vi "setposition.vi"(1 "Vy":dbl, 2 "Vx":dbl) -> ()   [LabVIEW 2015]
uses:
  <vilib>/DAQmx/write.llb/DAQmx Write (Analog 1D DBL NChan 1Samp).vi
  <vilib>/DAQmx/create/channels.llb/DAQmx Create Channel (AO-Voltage-Basic).vi
  <vilib>/DAQmx/miscellaneous.llb/DAQmx Fill In Error Info.vi
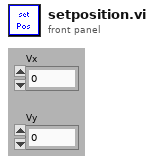
[diagram p1: front panel]
types:
  T1 = typedef "XYZStage.lvlib/XYZStage Configuration.ctl" = cluster{"VISA resource name":refnum<visa-resource-name>, "Timeout (3sec)":u32}
  T2 = cluster{"StageS":i32, "StageL":i32, "currmeas data dir":path, "image OD":u16, "contour OD":u16, "point OD":u16, "AOlines":tag[], "AIlines":tag[], "CI lines":tag[], "DO lines":tag[], "AO names":string[], "CI names":string[], "AI names":string[], "DO names":string[], "CIextensions":string[], "AIextensions":string[], "Voltage to Ygalvo":i32, "Voltage to Xgalvo":i32, "Voltage to patch":i32, "640 shutter":i32, "2P shutter":i32, "LT timestamp":u32, "Vp":i32, "Ip":i32, "camera trigger":i32, "master data dir":path, "voltage to Zpos":i32, "Vto2P":i32, "640 AO":i32, "488 AO":i32, "532 AO":i32, "640TTL":u32, "488TTL":u32, "532TTL":u32, "Device 1 sampleclock out":tag, "Device 1 Starttrigger out":tag, "Device 2 sampleclock in":tag, "Device 2 StartTrigger in ":tag, "2PODTTL":u32, "488 shutter":u32, "LCVR red":u32, "LCVR blue":u32, "Sutter Stage Config":T1, "Device 1 ext sampleclock in (100Khz)":tag}
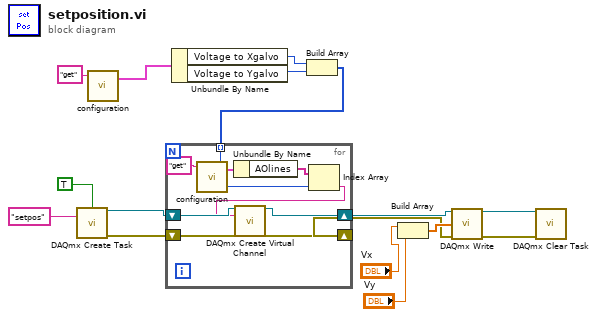
[diagram p0: block diagram]
diagram:
  n1 = call <vilib>:"DAQmx Create Task.vi"("new task name"="setpos", "auto cleanup"=TRUE) -> ("task out"=w10:refnum<k21>, "error out"=w8:errorcluster)  [unwired: 12 in]
  n2 = call "configuration.vi"("command"="get") -> ("config out"=w4:T2)  [unwired: 2 in, 1 out]
  n3 = Unbundle By Name(w4) -> ("Voltage to Xgalvo"=w3:i32, "Voltage to Ygalvo"=w2:i32)
  n4 = Build Array(w3, w2) -> (w1:i32[])
  n5 = for {
    shift-right: [w25] -> w11
    shift-left: w10 -> [w24]
    shift-right: [w22] -> w7
    shift-left: w8 -> [w23]
    tunnel: w1 -> [w19] mode=indexing
    n6 = call "configuration.vi"("command"="get") -> ("config out"=w20:T2)  [unwired: 2 in, 1 out]
    n7 = Unbundle By Name(w20) -> ("AOlines"=w18:tag[])
    n8 = Index Array(array=w18, index=w19) -> (element=w17:tag)
    n9 = call-poly <vilib>:"DAQmx Create Virtual Channel.vi"("task in"=w24, "physical channels"=w17, "error in"=w23) -> ("task out"=w25:refnum<k21>, "error out"=w22:errorcluster)  [unwired: 11 in]
  }
  n10 = Build Array("Vx", "Vy") -> (w12:dbl[])
  n11 = call-poly <vilib>:"DAQmx Write.vi"("task/channels in"=w11, "data"=w12, "error in"=w7) -> ("task out"=w13:refnum<k21>, "error out"=w14:errorcluster)  [unwired: 10 in, 1 out]
  n12 = call <vilib>:"DAQmx Clear Task.vi"("task in"=w13, "error in"=w14) -> ()  [unwired: 14 out]
